vi "Read CellData.vi"(8 "error in":errorcluster, 11 "CRDS Data in":refnum<class "CRDS Data.lvclass">) -> (0 "error out":errorcluster, 2 "CellData":refnum<class "CRDS Cell Data.lvclass">[](array[class]), 3 "CRDS Data out":refnum<class "CRDS Data.lvclass">)   [LabVIEW 2015, in "CRDS Lib.lvlib" / "CRDS Data.lvclass"]
doc: "Retrieve all data stored in the CRDS Cell Data class, an array of objects associated with the CRDS Data class. These objects store the data associated with each cell."
uses:
  CRDS Data.lvclass
  Cell/CRDS Cell Data.lvclass
  CRDS Data.lvclass/CRDS Data.ctl
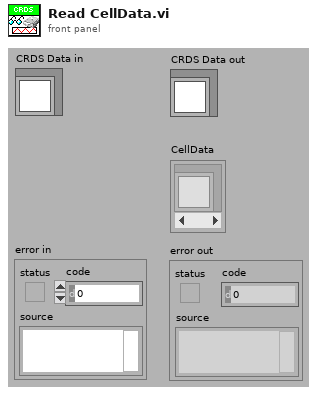
[diagram p1: front panel]
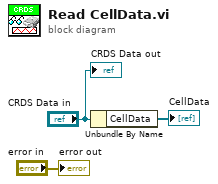
[diagram p0: block diagram]
diagram:
  n1 = Unbundle By Name("CRDS Data in") -> ("CellData"=→"CellData":refnum<class "CRDS Cell Data.lvclass">[])
  "error out" <- "error in"
  "CRDS Data out" <- "CRDS Data in"
